vi "NMR_Long_RF_Pulse_Sequence_V6.vi"() -> ()   [LabVIEW 2020]
uses:
  <instrlib>/niFgen/niFgen.llb/niFgen Output Mode.ctl
  <instrlib>/niFgen/niFgen.llb/niFgen Waveform Type.ctl
  <instrlib>/niFgen/niFgen.llb/niFgen_ctl Trigger DigEdge - Edge Values (Ring).ctl
  <instrlib>/niFgen/niFgen.llb/niFgen_ctl Trigger Source Values (Ring).ctl
  <instrlib>/niFgen/niFgen.llb/niFgen Trigger Mode.ctl
  <instrlib>/niScope/Controls/niScope acquisition type.ctl
  <instrlib>/niScope/Controls/niScope trigger slope.ctl
  <instrlib>/niScope/Controls/niScope trigger source.ctl
  <vilib>/Analysis/2dsp.llb/Integral Method.ctl
  <vilib>/Analysis/8numeric.llb/1D Numeric Integration.vi
  <vilib>/Utility/file.llb/Read Delimited Spreadsheet (DBL).vi
  <instrlib>/niFgen/niFgen.llb/niFgen Create Waveform (DBL).vi
  <instrlib>/niScope/Configure/Trigger/niScope Configure Trigger Edge.vi
  <instrlib>/niFgen/niFgen.llb/niFgen Configure Digital Edge Start Trigger.vi
  <instrlib>/niScope/Acquire/Fetch/niScope Fetch Cluster.vi
  <vilib>/Waveform/WDTFileIO.llb/Export Waveform To Spreadsheet File.vi
  <vilib>/Analysis/NI_AALPro.lvlib
panel:
  out "Averaged T2 Decay":waveform(dbl)(graph)={"t0"=timestamp(0 s since 1904-01-01), "dt"=0.0025142857142857146, "Y"=array[865 elements]} caption="Waveform Graph"
  out "Pulse Echos - Current Scan":T1(graph) caption="Waveform Graph"
  in  "Write Output to File?":bool
  out "Scan Number":i32=1
  out "Signal Intensity (Integral)":dbl=0.2866310909595196 format="%0.4f"
  out "Extracted T2 Decay - Current Scan":waveform(dbl)(graph)={"t0"=timestamp(0 s since 1904-01-01), "dt"=0.0025142857142857146, "Y"=array[865 elements]} caption="Waveform Graph"
  in  "Pulse Train File":path=path "D:/Pulse Train - 5s Duration, 3965 Pulses, 1.25ms Tau.txt"
  in  "Larmor Frequency":dbl=27457000.0 caption="Frequency" format="%.4p"
  in  "Number of Scans":i32=32
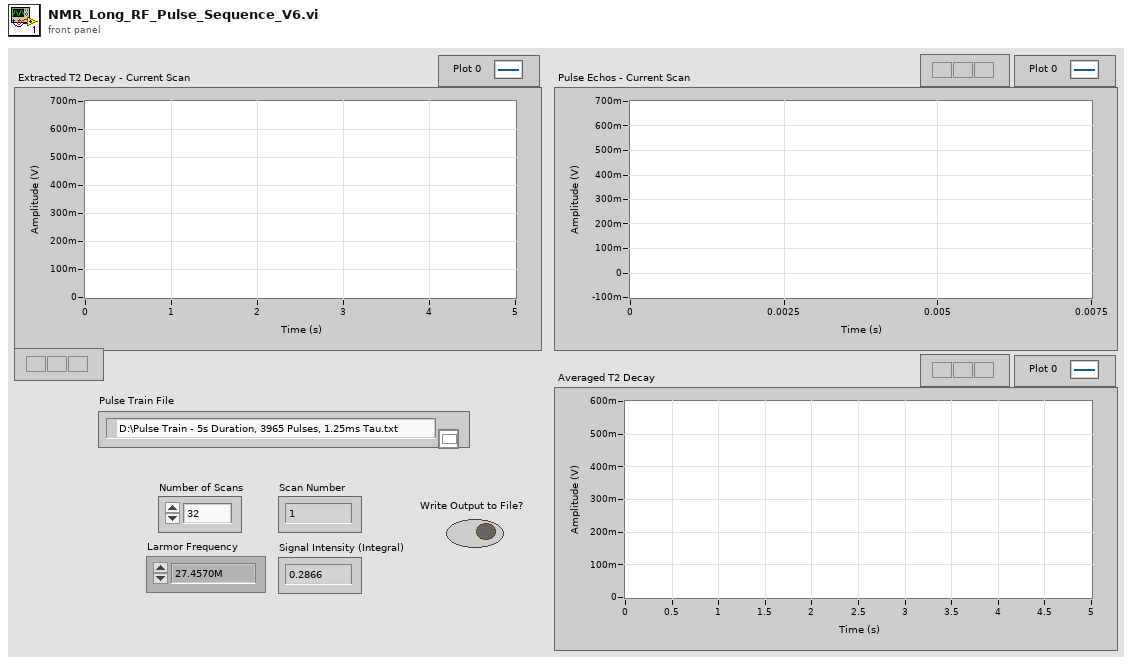
[diagram p1: front panel]
types:
  T1 = cluster{"relativeInitialX":dbl, "xIncrement":dbl, "wfm":dbl[]}
  T2 = typedef "niFgen Output Mode.ctl" = u32
  T3 = typedef "niScope trigger source.ctl" = string
  T4 = typedef "niFgen_ctl Trigger Source Values (Ring).ctl" = string
  T5 = typedef "NI_AALPro.lvlib/Integral Method.ctl" = i32
  T6 = typedef "niScope trigger slope.ctl" = i32
  T7 = typedef "niScope acquisition type.ctl" = i32
  T8 = typedef "niFgen Trigger Mode.ctl" = i32
  T9 = typedef "niFgen_ctl Trigger DigEdge - Edge Values (Ring).ctl" = i32
  T10 = typedef "niFgen Waveform Type.ctl" = i32
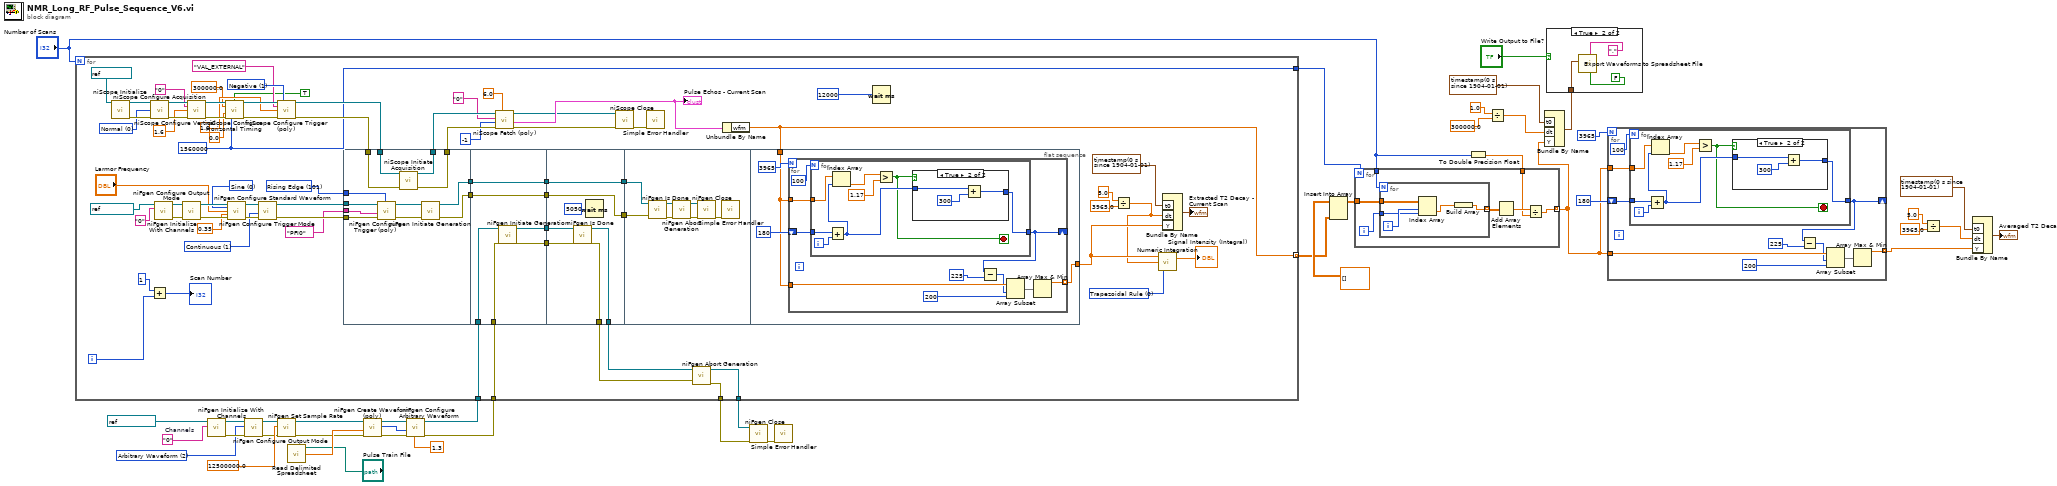
[diagram p0: block diagram]
diagram:
  w28 = "0"  # Channels
  w27 = T2 2 items=["Standard Function", "Frequency List", "Arbitrary Waveform", "Arbitrary Sequence", "Script"] ("output mode")
  n1 = call <instrlib>:"niFgen Initialize With Channels.vi"("Channel Name"=w28, "Resource Name"=refnum<k15> "PulseTrain" ("FGEN Resource Name 2")) -> ("error out"=w31:errorcluster, "Instrument Handle Out"=w32:refnum<k15>)  [unwired: 8 in]
  n2 = call <instrlib>:"niFgen Configure Output Mode.vi"("error in (no error)"=w31, "Output Mode (default: 0=Standard Function)"=w27, "Instrument Handle"=w32) -> ("error out"=w35:errorcluster, "Instrument Handle Out"=w34:refnum<k15>)  [unwired: 6 in]
  n3 = call <instrlib>:"niFgen Set Sample Rate.vi"("error in (no error)"=w35, "Sample Rate (Samp/s)"=12500000.0 ("Sample Rate"), "Instrument Handle"=w34) -> ("error out"=w38:errorcluster, "Instrument Handle Out"=w37:refnum<k15>)  [unwired: 7 in]
  n4 = call-poly <vilib>:"Read Delimited Spreadsheet.vi"("file path (dialog if empty)"="Pulse Train File") -> ("first row"=w39:dbl[])  [unwired: 9 in, 5 out]
  n5 = call-poly <instrlib>:"niFgen Create Waveform (poly).vi"("error in (no error)"=w38, "Waveform Data Array"=w39, "Instrument Handle"=w37) -> ("error out"=w41:errorcluster, "Waveform Handle"=w42:i32, "Instrument Handle Out"=w40:refnum<k15>)  [unwired: 6 in]
  n6 = call <instrlib>:"niFgen Configure Arbitrary Waveform.vi"("Gain"=1.3, "error in (no error)"=w41, "Waveform Handle"=w42, "Instrument Handle"=w40) -> ("error out"=w26:errorcluster, "Instrument Handle Out"=w25:refnum<k15>)  [unwired: 6 in]
  n7 = for {
    N: "Number of Scans" -> [_]
    tunnel: w26 -> [w97]
    tunnel: w25 -> [w96]
    tunnel: [w95] -> w23
    tunnel: [w94] -> w22
    tunnel: [w48] -> w19 mode=indexing
    tunnel: [w43] -> w10
    i -> [w51]
    w53 = T5 0 items=["Trapezoidal Rule", "Simpson's Rule", "Simpson's 3/8 Rule", "Bode Rule"] ("integration method")
    w43 = 1560000 ("min record length")
    w82 = T6 1 items=["Positive", "Negative"] ("trigger slope")
    w83 = T7 0 items=["Normal"=0, "Flex Res"=1, "DDC"=3] ("acquisition Type")
    w102 = T8 1 items=["Single", "Continuous", "Stepped", "Burst"] ("Trigger Mode (default: 1=continuous)")
    w106 = T9 101 items=["Rising Edge"=101, "Falling Edge"=102] ("Edge (Rising)")
    w107 = T10 0 items=["Sine", "Square", "Triangle", "Ramp Up", "Ramp Down", "DC", "Noise", "User"] ("Waveform")
    n8 = call <instrlib>:"niScope Initialize.vi"("resource name"=refnum<k15> "OScope") -> ("instrument handle"=w84:refnum<k15>, "error out"=w85:errorcluster)  [unwired: 13 in]
    n9 = call <instrlib>:"niScope Configure Acquisition.vi"("instrument handle"=w84, "acquisition Type"=w83, "error in"=w85) -> ("instrument handle out"=w87:refnum<k15>, "error out"=w88:errorcluster)  [unwired: 11 in]
    n10 = Add(x=1, y=w51) -> (x+y=→"Scan Number":i32)
    n11 = call <instrlib>:"niFgen Initialize With Channels.vi"("Channel Name"="0", "Resource Name"=refnum<k15> "FuncGen" ("Sine Wave Module")) -> ("error out"=w112:errorcluster, "Instrument Handle Out"=w115:refnum<k15>)  [unwired: 8 in]
    n12 = call <instrlib>:"niFgen Configure Output Mode.vi"("error in (no error)"=w112, "Instrument Handle"=w115) -> ("error out"=w111:errorcluster, "Instrument Handle Out"=w114:refnum<k15>)  [unwired: 7 in]
    n13 = call <instrlib>:"niScope Configure Vertical.vi"("instrument handle"=w87, "channels"="0", "vertical range"=1.6, "error in"=w88) -> ("instrument handle out"=w89:refnum<k15>, "error out"=w90:errorcluster)  [unwired: 10 in]
    n14 = call <instrlib>:"niScope Configure Horizontal Timing.vi"("instrument handle"=w89, "enforce realtime"=TRUE, "min sample rate"=300000.0, "reference position"=0.0, "error in"=w90, "min record length"=w43) -> ("instrument handle out"=w91:refnum<k15>, "error out"=w92:errorcluster)  [unwired: 8 in]
    n15 = call <instrlib>:"niFgen Configure Standard Waveform.vi"("Instrument Handle"=w114, "Waveform"=w107, "Frequency"="Larmor Frequency", "Amplitude"=0.35, "error in (no error)"=w111) -> ("Instrument Handle Out"=w113:refnum<k15>, "error out"=w110:errorcluster)  [unwired: 9 in]
    n16 = call <instrlib>:"niFgen Configure Trigger Mode.vi"("error in (no error)"=w110, "Trigger Mode (default: 1=continuous)"=w102, "Instrument Handle"=w113) -> ("error out"=w105:errorcluster, "Instrument Handle Out"=w103:refnum<k15>)  [unwired: 7 in]
    n17 = call-poly <instrlib>:"niScope Configure Trigger (poly).vi"("instrument handle"=w91, "trigger slope"=w82, "trigger source"=T3 "VAL_EXTERNAL", "trigger level"=1.0, "error in"=w92) -> ("instrument handle out"=w76:refnum<k15>, "error out"=w75:errorcluster)  [unwired: 9 in]
    n18 = flat-sequence {
      tunnel: w106 -> [w126]
      tunnel: w105 -> [w125]
      tunnel: T4 "PFI0" ("Source") -> [w124]
      tunnel: w103 -> [w123]
      tunnel: w76 -> [w121]
      tunnel: w75 -> [w120]
      tunnel: [w119] -> w74
      tunnel: [w118] -> w73
      tunnel: [w117] -> w63
      tunnel: [w116] -> w60
      tunnel: w97 -> [w133]
      tunnel: w96 -> [w132]
      tunnel: [w131] -> w67
      tunnel: [w130] -> w66
      tunnel: [w129] -> w64
      tunnel: w63 -> [w129]
      tunnel: [w128] -> w61
      tunnel: w60 -> [w128]
      tunnel: [w139] -> w100
      tunnel: [w138] -> w99
      tunnel: w67 -> [w137]
      tunnel: w66 -> [w136]
      tunnel: [w135] -> w65
      tunnel: w64 -> [w135]
      tunnel: [w134] -> w62
      tunnel: w61 -> [w134]
      tunnel: w65 -> [w142]
      tunnel: w62 -> [w141]
      tunnel: w48 -> [w148]
      tunnel: [w150] -> w55
      frame #0 {
        n19 = call-poly <instrlib>:"niFgen Configure Trigger (poly).vi"("Edge (Rising)"=w126, "error in (no error)"=w125, "Source"=w124, "Instrument Handle"=w123) -> ("error out"=w122:errorcluster, "Instrument Handle Out"=w127:refnum<k15>)  [unwired: 6 in]
        n20 = call <instrlib>:"niScope Initiate Acquisition.vi"("instrument handle"=w121, "error in"=w120) -> ("instrument handle out"=w119:refnum<k15>, "error out"=w118:errorcluster)  [unwired: 12 in]
        n21 = call <instrlib>:"niFgen Initiate Generation.vi"("error in (no error)"=w122, "Instrument Handle"=w127) -> ("error out"=w116:errorcluster, "Instrument Handle Out"=w117:refnum<k15>)  [unwired: 8 in]
      }
      frame #1 {
        n22 = call <instrlib>:"niFgen Initiate Generation.vi"("error in (no error)"=w133, "Instrument Handle"=w132) -> ("error out"=w130:errorcluster, "Instrument Handle Out"=w131:refnum<k15>)  [unwired: 8 in]
      }
      frame #2 {
        n23 = call <instrlib>:"niFgen Is Done.vi"("error in (no error)"=w136, "Instrument Handle"=w137) -> ("error out"=w139:errorcluster, "Instrument Handle Out"=w138:refnum<k15>)  [unwired: 7 in, 1 out]
        n24 = Wait (ms)(milliseconds to wait=u32 5050) -> ()  [unwired: 1 out]
      }
      frame #3 {
        n25 = call <instrlib>:"niFgen Is Done.vi"("error in (no error)"=w141, "Instrument Handle"=w142) -> ("error out"=w145:errorcluster, "Instrument Handle Out"=w144:refnum<k15>)  [unwired: 7 in, 1 out]
        n26 = call <instrlib>:"niFgen Abort Generation.vi"("error in (no error)"=w145, "Instrument Handle"=w144) -> ("error out"=w146:errorcluster, "Instrument Handle Out"=w147:refnum<k15>)  [unwired: 8 in]
        n27 = call <instrlib>:"niFgen Close.vi"("error in (no error)"=w146, "Instrument Handle"=w147) -> ("error out"=w143:errorcluster)  [unwired: 9 in]
        n28 = call <vilib>:"Simple Error Handler.vi"("error in (no error)"=w143) -> ()  [unwired: 4 in, 5 out]
      }
      frame #4 {
        n29 = for {
          N: 3965 -> [_]
          tunnel: [w160] -> w150 mode=indexing
          tunnel: w148 -> [w159]
          shift-right: [w154] -> _
          shift-left: 180 -> [w155]
          tunnel: w148 -> [w153]
          n30 = for {
            N: 100 -> [_]
            tunnel: w153 -> [w165]
            tunnel: w155 -> [w168]
            tunnel: [w163] -> w154
            i -> [w169]
            stop <- w162 stop-if-true
            n31 = Add(x=w168, y=w169) -> (x+y=w164:i32)
            n32 = Index Array(array=w165, index=w164) -> (element=w166:dbl)
            n33 = Greater?(x=w166, y=1.17) -> (0:w162:bool)
            n34 = case shown="True" w162 {
              tunnel: w164 -> [w170 w171]
              tunnel: [w170 w173] -> w163
              frame False {
              }
              frame True {
                n35 = Add(x=w171, y=300) -> (x+y=w173:i32)
              }
            }
          }
          n36 = Subtract(x=w154, y=225) -> (x-y=w156:i32)
          n37 = Array Subset(array=w159, index=w156, length=200 ("y")) -> (w161:dbl[])
          n38 = Array Max & Min(array=w161) -> (max value=w160:dbl)  [unwired: 3 out]
        }
      }
    }
    n39 = call-poly <instrlib>:"niScope Fetch (poly).vi"("timeout"=6.0, "error in"=w73, "numSamples"=-1, "channels"="0", "instrument handle"=w74) -> ("error out"=w44:errorcluster, "waveform"=w47:T1, "instrument handle out"=w45:refnum<k15>)  [unwired: 3 in, 1 out]
    "Pulse Echos - Current Scan" <- w47
    n40 = call <instrlib>:"niScope Close.vi"("instrument handle"=w45, "error in"=w44) -> ("error out"=w93:errorcluster)  [unwired: 13 in]
    n41 = call <vilib>:"Simple Error Handler.vi"("error in (no error)"=w93) -> ()  [unwired: 4 in, 5 out]
    n42 = call <instrlib>:"niFgen Abort Generation.vi"("error in (no error)"=w100, "Instrument Handle"=w99) -> ("error out"=w95:errorcluster, "Instrument Handle Out"=w94:refnum<k15>)  [unwired: 8 in]
    n43 = Unbundle By Name(w47) -> ("wfm"=w48:dbl[])
    n44 = Wait (ms)(milliseconds to wait=u32 12000 ("Delay Time (ms)")) -> ()  [unwired: 1 out]
    n45 = Divide(x=5.0, y=3965.0) -> (x/y=w54:dbl)
    n46 = call-poly <vilib>:"Numeric Integration.vi"("integration method"=w53, "dt"=w54, "Input Array"=w55) -> ("result"=→"Signal Intensity (Integral)":dbl)  [unwired: 1 out]
    n47 = Bundle By Name("t0"=timestamp(0 s since 1904-01-01), "dt"=w54, "Y"=w55) -> (→"Extracted T2 Decay - Current Scan":waveform(dbl))  [unwired: 1 in]
  }
  n48 = call <instrlib>:"niFgen Close.vi"("error in (no error)"=w23, "Instrument Handle"=w22) -> ("error out"=w24:errorcluster)  [unwired: 9 in]
  n49 = call <vilib>:"Simple Error Handler.vi"("error in (no error)"=w24) -> ()  [unwired: 4 in, 5 out]
  n50 = Insert Into Array(array=dbl[][] [], new element=w19) -> (w21:dbl[][])  [unwired: 2 in]
  n51 = To Double Precision Float(number="Number of Scans") -> (double precision float=w18:dbl)
  n52 = for {
    N: w10 -> [_]
    tunnel: w21 -> [w180]
    tunnel: [w176] -> w2 mode=indexing
    tunnel: "Number of Scans" -> [w175]
    tunnel: w18 -> [w174]
    i -> [w179]
    n53 = for {
      N: w175 -> [_]
      tunnel: w180 -> [w185]
      tunnel: w179 -> [w183]
      tunnel: [w181] -> w178 mode=indexing
      i -> [w184]
      n54 = Index Array(array=w185, index (row)=w184, index (col)=w183) -> (element=w182:dbl)
      n55 = Build Array(w182) -> (w181:dbl[])
    }
    n56 = Add Array Elements(numeric array=w178) -> (sum=w177:dbl)
    n57 = Divide(x=w177, y=w174) -> (x/y=w176:dbl)
  }
  n58 = Divide(x=1.0, y=300000.0) -> (x/y=w13:dbl)
  n59 = Bundle By Name("t0"=timestamp(0 s since 1904-01-01), "dt"=w13, "Y"=w2) -> (w12:waveform(dbl))  [unwired: 1 in]
  n60 = case shown="True" "Write Output to File?" {
    tunnel: w12 -> [_ w186]
    frame False {
    }
    frame True {
      n61 = call-poly <vilib>:"Export Waveforms to Spreadsheet File.vi"("header? (write header:T)"=FALSE, "delimiter (Tab)"=",", "waveform"=w186) -> ()  [unwired: 7 in, 2 out]
    }
  }
  n62 = for {
    N: 3965 -> [_]
    tunnel: [w197] -> w1 mode=indexing
    tunnel: w2 -> [w196]
    shift-right: [w191] -> _
    shift-left: 180 -> [w192]
    tunnel: w2 -> [w190]
    n63 = for {
      N: 100 -> [_]
      tunnel: w190 -> [w202]
      tunnel: w192 -> [w205]
      tunnel: [w200] -> w191
      i -> [w206]
      stop <- w199 stop-if-true
      n64 = Add(x=w205, y=w206) -> (x+y=w201:i32)
      n65 = Index Array(array=w202, index=w201) -> (element=w203:dbl)
      n66 = Greater?(x=w203, y=1.17) -> (0:w199:bool)
      n67 = case shown="True" w199 {
        tunnel: w201 -> [w207 w208]
        tunnel: [w207 w210] -> w200
        frame False {
        }
        frame True {
          n68 = Add(x=w208, y=300) -> (x+y=w210:i32)
        }
      }
    }
    n69 = Subtract(x=w191, y=225) -> (x-y=w193:i32)
    n70 = Array Subset(array=w196, index=w193, length=200 ("y")) -> (w198:dbl[])
    n71 = Array Max & Min(array=w198) -> (max value=w197:dbl)  [unwired: 3 out]
  }
  n72 = Divide(x=5.0, y=3965.0) -> (x/y=w5:dbl)
  n73 = Bundle By Name("t0"=timestamp(0 s since 1904-01-01), "dt"=w5, "Y"=w1) -> (→"Averaged T2 Decay":waveform(dbl))  [unwired: 1 in]
